vi "Shutdown Main.vi"(8 "error out":errorcluster) -> ()   [LabVIEW 2014]
uses:
  Aircraft Information/Sub VI/Get Aircraft Information.vi
  Ground Station to Aircraft Coms/SubVI/Aircraft Data Router/SubVI/Queue References/SubVI/Get Aircraft TX Queue String.vi
  Ground Station to Aircraft Coms/SubVI/Aircraft Data Router/SubVI/Queue References/SubVI/Get Aircraft RX Queue String.vi
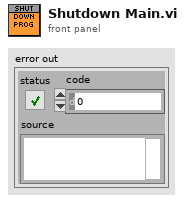
[diagram p1: front panel]
types:
  T1 = typedef "Drone Information.ctl" = cluster{"Heart Beat":bool, "Aircraft ID":u8, "Downlink Port":refnum<visa-resource-name>, "Tag ID":string, "System Status":string, "Base Mode":T2, "Armed/Disarmed":bool, "Battery Voltage":dbl, "Control Mode":T3, "Initialisation":u8, "Heart Beat Status":bool, "Uplink Port":refnum<visa-resource-name>, "UDP connection ID":refnum<k16>, "Connection Type":T4, "Mode":string, "UDP IP Address":string, "Mission Uploaded":bool}
  T2 = typedef "Base Mode.ctl" = cluster{"Custom Mode":bool, "Test Enabled":bool, "Autonomous Mode":bool, "Guided Mode":bool, "Stabilization Enabled":bool, "HIL Enabled":bool, "Manual Mode":bool, "Arm":bool}
  T3 = typedef "Aircraft Mode.ctl" = enum16{"Loiter", "Stabalise", "Failsafe", "Emergency Stop"}
  T4 = typedef "Telemetry Connection Type.ctl" = enum16{"Serial", "UDP", "TCP"}
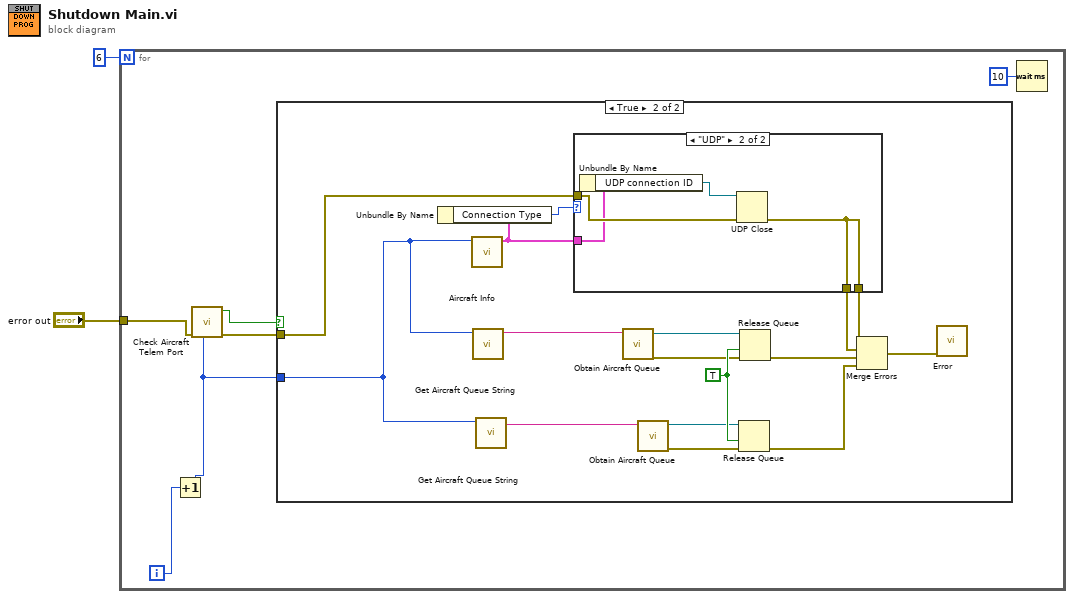
[diagram p0: block diagram]
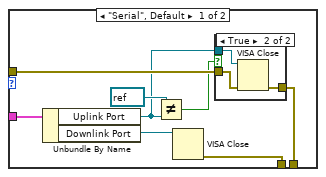
[diagram p3: hidden frame]
diagram:
  n1 = for {
    N: 6 -> [_]
    tunnel: "error out" -> [w7]
    i -> [w5]
    n2 = Increment(x=w5) -> (x+1=w4:i32)
    n3 = call "Check Aircraft Telem Port.vi"("Error In"=w7, "Aircraft ID"=w4) -> ("Error Out"=w3:errorcluster, "Telem Port Found"=w6:bool)  [unwired: 8 in]
    n4 = case shown="True" w6 {
      tunnel: w4 -> [_ w13]
      tunnel: w3 -> [_ w12]
      frame False {
      }
      frame True {
        w24 = TRUE ("force destroy? (F)")
        n5 = call-poly "Aircraft Info.vi"("Aircraft ID"=w13) -> ("Aircraft Information Out"=w10:T1)  [unwired: 9 in, 1 out]
        n6 = Unbundle By Name(w10) -> ("Connection Type"=w9:T4)
        n7 = call-poly "Get Aircraft Queue String.vi"("Aircraft ID"=w13) -> ("Aircraft Q Name"=w21:string)  [unwired: 9 in, 1 out]
        n8 = call-poly "Get Aircraft Queue String.vi"("Aircraft ID"=w13) -> ("Aircraft Queue Name"=w18:string)  [unwired: 9 in, 1 out]
        n9 = case shown="\"UDP\"" w9 {
          tunnel: w10 -> [w32 w39]
          tunnel: [w30 w37] -> w17
          tunnel: w12 -> [w29 w40]
          tunnel: [w28 w37] -> w11
          frame "Serial", Default {
            n10 = Unbundle By Name(w32) -> ("Uplink Port"=w25:refnum<visa-resource-name>, "Downlink Port"=w31:refnum<visa-resource-name>)
            n11 = Not Equal?(x=refnum<visa-resource-name> refnum, y=w25) -> (x != y?=w26:bool)
            n12 = VISA Close(VISA resource name=w31) -> (error out=w30:errorcluster)  [unwired: 1 in]
            n13 = case shown="True" w26 {
              tunnel: w29 -> [w33 w36]
              tunnel: [w33 w35] -> w28
              tunnel: w25 -> [_ w34]
              frame False {
              }
              frame True {
                n14 = VISA Close(VISA resource name=w34, error in (no error)=w36) -> (error out=w35:errorcluster)
              }
            }
          }
          frame "UDP" {
            n15 = Unbundle By Name(w39) -> ("UDP connection ID"=w38:refnum<k16>)
            n16 = UDP Close(connection ID=w38, 8:w40) -> (error out=w37:errorcluster)  [unwired: 1 out]
          }
        }
        n17 = call "Obtain Aircraft Queue.vi"("Queue Name"=w21) -> ("error out"=w23:errorcluster, "queue out"=w22:refnum<queue>)  [unwired: 9 in]
        n18 = call "Obtain Aircraft Queue.vi"("Queue Name"=w18) -> ("error out"=w19:errorcluster, "queue out"=w20:refnum<queue>)  [unwired: 9 in]
        n19 = Release Queue(queue=w20, force destroy? (F)=w24, error in (no error)=w19) -> (error out=w15:errorcluster)  [unwired: 2 out]
        n20 = Release Queue(queue=w22, force destroy? (F)=w24, error in (no error)=w23) -> (error out=w16:errorcluster)  [unwired: 2 out]
        n21 = Merge Errors(w11, w17, w16, w15) -> (w14:errorcluster)
        n22 = call "Error.vi"("Error In"=w14) -> ()  [unwired: 10 in, 1 out]
      }
    }
    n23 = Wait (ms)(milliseconds to wait=u32 10) -> ()  [unwired: 1 out]
  }
